vi "My OWn PID Gyro.vi"(8 "Current Input":dbl, 10 "Wanted End":dbl, 11 "Negate Stuff":bool) -> (2 "Output":dbl, 3 "Done":bool)   [LabVIEW 2017]
uses:
  <vilib>/Rock Robotics/Network Tables/NT Write Number.vi
panel:
  # "determines what way to turn"
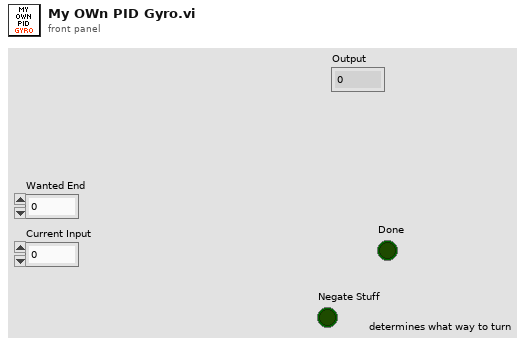
[diagram p1: front panel]
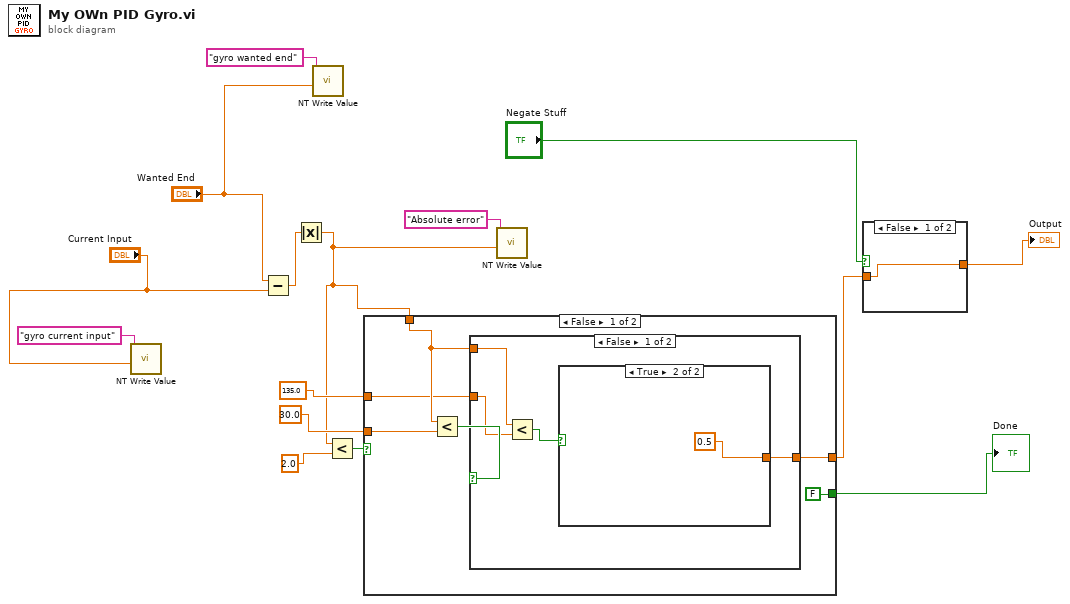
[diagram p0: block diagram]
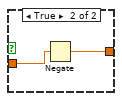
[diagram p2: hidden frame]
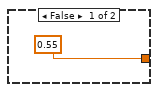
[diagram p3: hidden frame]
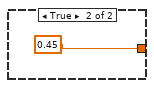
[diagram p4: hidden frame]
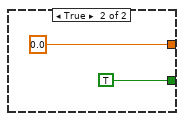
[diagram p5: hidden frame]
diagram:
  n1 = call-poly <vilib>:"NT Write Value.vi"("Numeric"="Current Input", "Name"="gyro current input") -> ()  [unwired: 9 in, 1 out]
  n2 = Subtract(x="Wanted End", y="Current Input") -> (x-y=w13:dbl)
  n3 = Absolute Value(x=w13) -> (abs(x)=w2:dbl)
  n4 = call-poly <vilib>:"NT Write Value.vi"("Numeric"="Wanted End", "Name"="gyro wanted end") -> ()  [unwired: 9 in, 1 out]
  n5 = Less?(x=w2, y=2.0) -> (x < y?=w15:bool)
  n6 = case shown="False" w15 {
    tunnel: w2 -> [w18 _]
    tunnel: [w19 0.0] -> w14
    tunnel: 30.0 -> [w21 _]
    tunnel: 135.0 -> [w17 _]
    tunnel: [FALSE TRUE] -> w8
    frame False {
      n7 = Less?(x=w18, y=w21) -> (x < y?=w20:bool)
      n8 = case shown="False" w20 {
        tunnel: [w23 0.45] -> w19
        tunnel: w18 -> [w25 _]
        tunnel: w17 -> [w24 _]
        frame False {
          n9 = Less?(x=w25, y=w24) -> (x < y?=w22:bool)
          n10 = case shown="True" w22 {
            tunnel: [0.55 0.5] -> w23
            frame False {
            }
            frame True {
            }
          }
        }
        frame True {
        }
      }
    }
    frame True {
    }
  }
  "Done" <- w8
  n11 = call-poly <vilib>:"NT Write Value.vi"("Numeric"=w2, "Name"="Absolute error") -> ()  [unwired: 9 in, 1 out]
  n12 = case shown="False" "Negate Stuff" {
    tunnel: w14 -> [w31 w33]
    tunnel: [w31 w32] -> w12
    frame False {
    }
    frame True {
      n13 = Negate(x=w33) -> (-x=w32:dbl)
    }
  }
  "Output" <- w12
